vi "SNTguiver1.vi"() -> ()   [LabVIEW 2020]
uses:
  EventController.ctl
panel:
  in  "Submit":bool
  in  "Seal Start Test":bool
  in  "Leak Start Test":bool
  in  "Start Testing":bool
  out "Event":dbl
  in  "stop":bool
  in  "Back":bool
  out "Results":string
  in  "Battery ID:":string
  out "User Allowed":bool
  in  "CHECK":bool
  in  "Badge #:":string
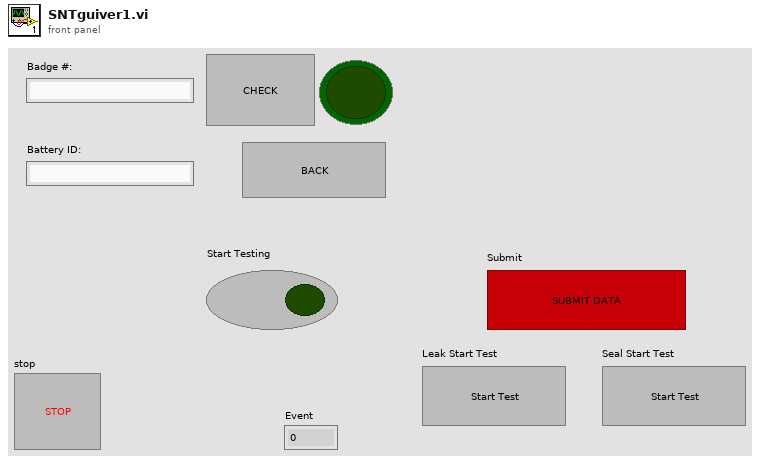
[diagram p1: front panel]
types:
  T1 = typedef "EventController.ctl" = enum16{"Idle", "Privilege", "Testing", "Submit"}
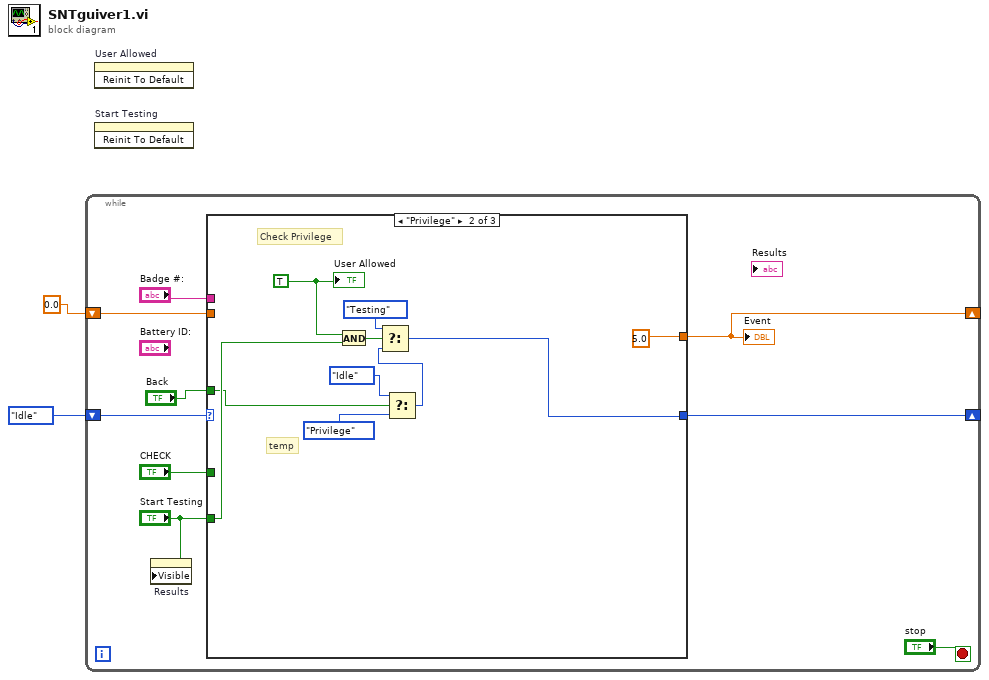
[diagram p0: block diagram]
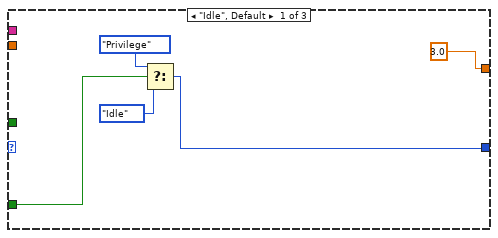
[diagram p2: hidden frame]
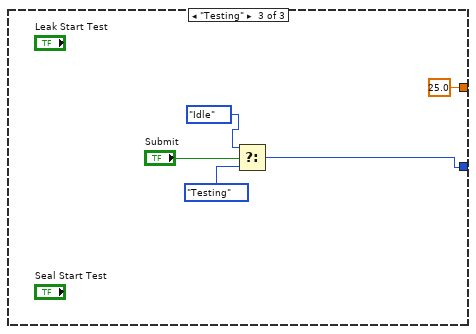
[diagram p3: hidden frame]
diagram:
  n1 = while {
    shift-right: [w10] -> _
    shift-left: EventController."Idle" -> [w11]
    shift-right: [w5] -> _
    shift-left: 0.0 -> [w6]
    stop <- "stop" stop-if-true
    n2 = property on="Results" class="Str"("Visible"="Start Testing") -> ()  [unwired: 2 in, 2 out]
    n3 = case shown="\"Privilege\"" w11 {
      tunnel: [w12 w18 w27] -> w10
      tunnel: "CHECK" -> [w16 _ _]
      tunnel: "Badge #:" -> [_ _ _]
      tunnel: [3.0 5.0 25.0] -> w5
      tunnel: w6 -> [_ _ _]
      tunnel: "Start Testing" -> [_ w21 _]
      tunnel: "Back" -> [_ w17 _]
      frame "Idle", Default {
        n4 = Select(t=EventController."Privilege", s=w16, f=EventController."Idle") -> (s? t:f=w12:T1)
      }
      frame "Privilege" {
        w22 = TRUE
        # "temp"
        # "Check Privilege"
        n5 = And(x=w22, y=w21) -> (x .and. y?=w23:bool)
        n6 = Select(t=EventController."Idle", s=w17, f=EventController."Privilege") -> (s? t:f=w19:T1)
        n7 = Select(t=EventController."Testing", s=w23, f=w19) -> (s? t:f=w18:T1)
        "User Allowed" <- w22
      }
      frame "Testing" {
        n8 = Select(t=EventController."Idle", s="Submit", f=EventController."Testing") -> (s? t:f=w27:T1)
      }
    }
    "Event" <- w5
  }
  n9 = invoke on="User Allowed" class="Bool (strict)" method="Reinit To Default"() -> ()  [unwired: 3 in, 3 out]
  n10 = invoke on="Start Testing" class="Bool (strict)" method="Reinit To Default"() -> ()  [unwired: 3 in, 3 out]
